vi "Validate Sample Period.vi"(1 "Sample Period (msec)":i32) -> (0 "Result":T1)   [LabVIEW 2015, in "Config Data.lvlib" / "Config Data.lvclass"]
uses:
  Config Data.lvclass
  Startup Processes/_typedefs/Data Valid Flag.ctl
  Startup Processes/Startup Processes.lvlib
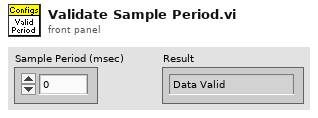
[diagram p1: front panel]
types:
  T1 = typedef "Startup Processes.lvlib/Data Valid Flag.ctl" = enum16{"Data Valid", "Data Not Valid"}
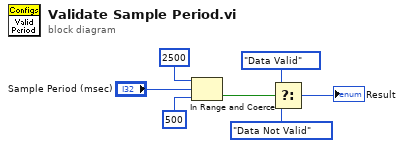
[diagram p0: block diagram]
diagram:
  n1 = In Range and Coerce(upper limit=2500, x="Sample Period (msec)", lower limit=500 ("upper limit")) -> (In Range?=w5:bool)  [unwired: 1 out]
  n2 = Select(t=Data_Valid_Flag."Data Valid" ("Enum"), s=w5, f=Data_Valid_Flag."Data Not Valid" ("Enum")) -> (s? t:f=→"Result":T1)
